vi "Bool To Disabled.vi"(1 "Bool":bool) -> (0 "Disabled":T1(ring)=enum."Disabled and Grayed Out")   [LabVIEW 2019]
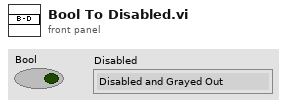
[diagram p1: front panel]
types:
  T1 = enum8{"Enabled", "Disabled", "Disabled and Grayed Out"}
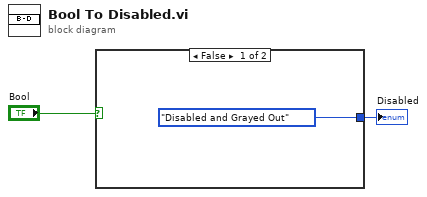
[diagram p0: block diagram]
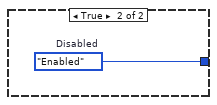
[diagram p2: hidden frame]
diagram:
  n1 = case shown="False" "Bool" {
    tunnel: [T1."Disabled and Grayed Out" ("Disabled") w4] -> w1
    frame False {
    }
    frame True {
      w4 = T1."Enabled"  # Disabled
    }
  }
  "Disabled" <- w1
